vi "Count occurrences in string.vi"(2 "Input string":string, 3 "Expression":string) -> (14 "Occurrences":i32)   [LabVIEW 2026]
doc: "This VI counts, how often an expression occurs in a string."
panel:
  # "This vi counts, how often an expression \noccurs in a string."
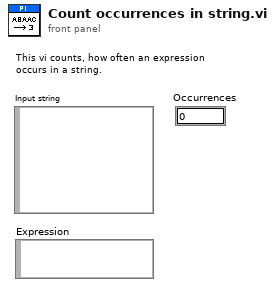
[diagram p1: front panel]
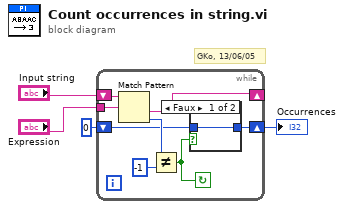
[diagram p0: block diagram]
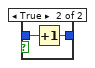
[diagram p2: hidden frame]
diagram:
  # "GKo, 13/06/05"
  n1 = while {
    tunnel: "Expression" -> [w6]
    shift-left: "Input string" -> [w7]
    shift-right: [w5] -> _
    shift-left: 0 -> [w8]
    shift-right: [w9] -> w1
    stop <- w12 continue-if-true
    n2 = Match Pattern(string=w7, regular expression=w6) -> (after substring=w5:string, offset past match=w10:i32)  [unwired: 3 out]
    n3 = Not Equal?(x=w10, y=-1) -> (x != y?=w12:bool)
    n4 = case shown="Faux" w12 {
      tunnel: [w13 w15] -> w9
      tunnel: w8 -> [w13 w14]
      frame False {
      }
      frame True {
        n5 = Increment(x=w14) -> (x+1=w15:i32)
      }
    }
  }
  "Occurrences" <- w1
